vi "myRIO_BRig_RT_dataLC_Wrong_OnOff_l2.vi"() -> (2 "output_Wrong_OnOff_l2":i32)   [LabVIEW 2014]
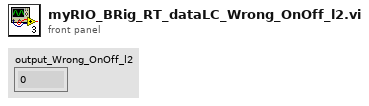
[diagram p1: front panel]
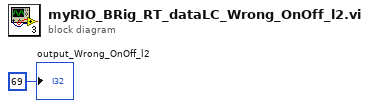
[diagram p0: block diagram]
diagram:
  "output_Wrong_OnOff_l2" <- 69 ("output_iBlock")
